vi "Actor Core.vi"(8 "error in":errorcluster, 11 "Pane Settings UI in":refnum<class "Pane Settings UI.lvclass">) -> (0 "error out":errorcluster, 3 "Actor out":refnum<class "Actor.lvclass">)   [LabVIEW 2015, in "Pane Settings UI.lvlib" / "Pane Settings UI.lvclass"]
doc: "The user interface for this panel.\n\n----\nPlease see the following web address for additional documentation and tutorial information:\nhttp://www.mooregoodideas.com/mgi-panel-manager/\n\nAuthor: Derek Trepanier\n\nCopyright (c) 2018, Moore Good Ideas, Inc.\n\nAll rights reserved.\n\nRedistribution and use in source and binary forms, with or without modification, are permitted provided that the following conditions are met:\n\n * Redistributions of source code must retain the above copyright notice, this list of conditions and the following disclaimer.\n * Redistributions in binary form must reproduce the above copyright notice, this list of conditions and the following disclaimer in the documentation and/or other materials provided with the distribution.\n * Neither the name of Moore Good Ideas, Inc. nor the names of its contributors may be used to endorse or promote products derived from this software without specific prior written permission.\n\nTHIS SOFTWARE IS PROVIDED BY THE COPYRIGHT HOLDERS AND CONTRIBUTORS \"AS IS\" AND ANY EXPRESS OR IMPLIED WARRANTIES, INCLUDING, BUT NOT LIMITED TO, THE IMPLIED WARRANTIES OF MERCHANTABILITY AND FITNESS FOR A PARTICULAR PURPOSE ARE DISCLAIMED. IN NO EVENT SHALL THE COPYRIGHT OWNER OR CONTRIBUTORS BE LIABLE FOR ANY DIRECT, INDIRECT, INCIDENTAL, SPECIAL, EXEMPLARY, OR CONSEQUENTIAL DAMAGES (INCLUDING, BUT NOT LIMITED TO, PROCUREMENT OF SUBSTITUTE GOODS OR SERVICES; LOSS OF USE, DATA, OR PROFITS; OR BUSINESS INTERRUPTION) HOWEVER CAUSED AND ON ANY THEORY OF LIABILITY, WHETHER IN CONTRACT, STRICT LIABILITY, OR TORT (INCLUDING NEGLIGENCE OR OTHERWISE) ARISING IN ANY WAY OUT OF THE USE OF THIS SOFTWARE, EVEN IF ADVISED OF THE POSSIBILITY OF SUCH DAMAGE."
uses:
  Pane Settings UI.lvclass
  <vilib>/ActorFramework/Actor/Actor.lvclass
  Typedefs/Point--Cluster.ctl
  Typedefs/Scrollbar Visibility--Enum.ctl
  Classes/Pane/Pane.lvclass
  <vilib>/ActorFramework/Actor/Actor.lvclass/Actor.ctl
  Pane Settings UI.lvclass/Pane Settings UI.ctl
  <vilib>/ActorFramework/Message Enqueuer/Message Enqueuer.lvclass/Message Enqueuer.ctl
  <vilib>/ActorFramework/Message Enqueuer/Enqueue.vi
  <vilib>/ActorFramework/Message Priority Queue/Priority Enqueue.vi
  Pane Relief Main UI/Pane Relief Main UI Messages/Panel Object Settings Changed Msg/Panel Object Settings Changed Msg.lvclass
  <vilib>/MGI/Panel Manager/Panel Actor/Panel Actor/Panel Actor.lvclass
panel:
  in  "Label":string
  in  "Set Min to Current":bool
  in  "Vertical Scroll":T1
  in  "Horizontal Scroll":T1 caption="Scrollbar"
  in  "Origin":T2
  in  "Min Pane":T2={"Horizontal"=1, "Vertical"=0} {"Vertical" min=0; "Horizontal" min=1}
  in  "Color":u32(colorbox)
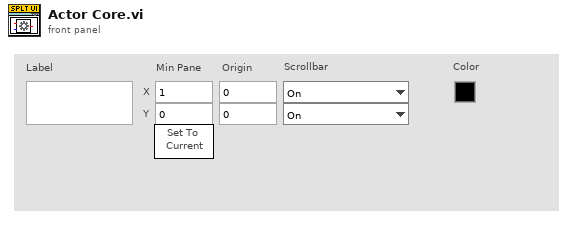
[diagram p1: front panel]
types:
  T1 = typedef "Scrollbar Visibility--Enum.ctl" = enum16{"On", "Off", "Off While Running"}
  T2 = typedef "Point--Cluster.ctl" = cluster{"Horizontal":i32, "Vertical":i32}
  T3 = cluster{"Event Registration Refnum":refnum<event-registration>, "Pnl Actor":refnum<event-registration>}
  T4 = typedef "LVPointTypeDef.ctl" = cluster{"Horizontal":i16, "Vertical":i16}
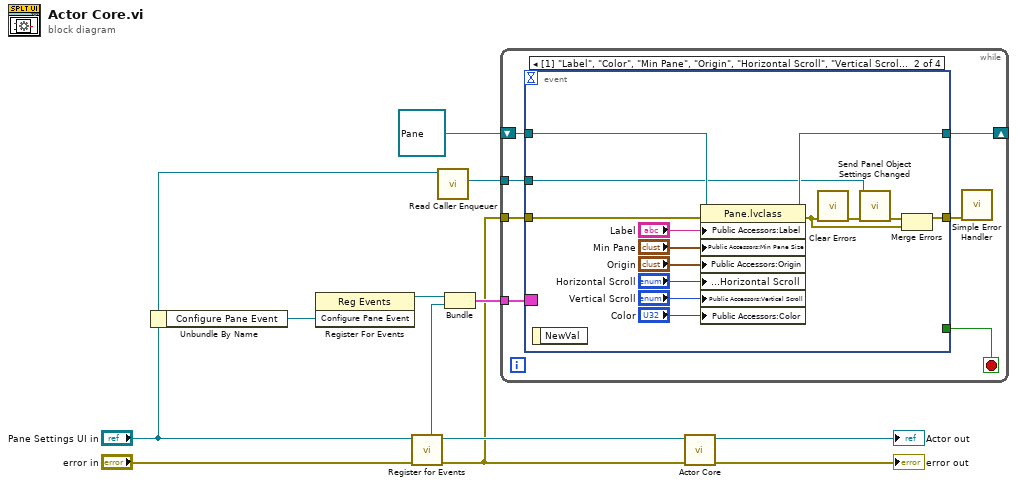
[diagram p0: block diagram]
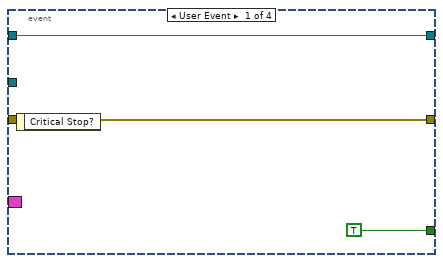
[diagram p2: hidden frame]
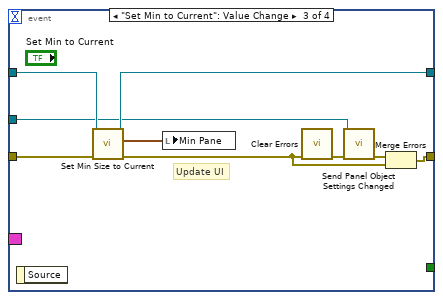
[diagram p3: hidden frame]
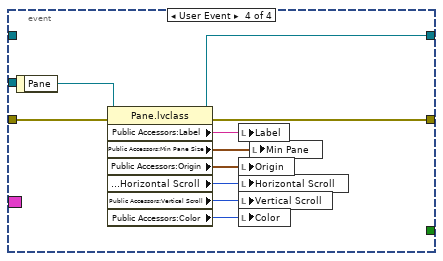
[diagram p4: hidden frame]
diagram:
  n1 = Unbundle By Name("Pane Settings UI in") -> ("Configure Pane Event"=w1:refnum<user-event>)
  n2 = register-events(w1) -> (reference out=w8:refnum<event-registration>)  [unwired: 2 in, 1 out]
  n3 = call <vilib>:"Register for Events.vi"("Error In"="error in", "Panel Actor in"="Pane Settings UI in") -> ("Error Out"=w4:errorcluster, "Panel Actor out"=w10:refnum<class "Pane Settings UI.lvclass">, "Pnl Actor"=w7:refnum<event-registration>)  [unwired: 6 in, 1 out]
  n4 = call <vilib>:"Read Caller Enqueuer.vi"("Actor"="Pane Settings UI in") -> ("Caller Enqueuer"=w3:refnum<class "Message Enqueuer.lvclass">)  [unwired: 10 in]
  n5 = Bundle("Event Registration Refnum"=w8, "Pnl Actor"=w7) -> (w6:T3)  [unwired: 1 in]
  n6 = while {
    tunnel: w6 -> [w19]
    shift-right: [w17] -> _
    shift-left: refnum<class "Pane.lvclass"> refnum ("Pane.lvclass") -> [w16]
    tunnel: w3 -> [w14]
    tunnel: w4 -> [w15]
    stop <- w18 stop-if-true
    n7 = event shown="[1] \"Label\", \"Color\", \"Min Pane\", \"Origin\", \"Horizontal Scroll\", \"Vertical Scroll\": Value Change" {
      selector: w19 -> [_ _ _ _]
      dyn-events: _ -> [_ _ _ _]
      timeout: _ -> [_ _ _ _]
      tunnel: [TRUE _ _ _] -> w18
      tunnel: [w21 w29 w43 w53] -> w17
      tunnel: w16 -> [w21 w28 w44 _]
      tunnel: w15 -> [w20 w36 w45 w55]
      tunnel: [w20 w25 w38 w54] -> w13
      tunnel: w14 -> [_ w23 w37 _]
      event User Event {
        n8 = event-data() -> ()  [unwired: 1 in, 1 out]
      }
      event "Label", "Color": Value Change {
        n9 = event-data() -> ()  [unwired: 1 in, 1 out]
        n10 = property class="Pane.lvclass"(reference=w28, error in=w36, "Public Accessors:Label"="Label", "Public Accessors:Min Pane Size"="Min Pane", "Public Accessors:Origin"="Origin", "Public Accessors:Horizontal Scroll"="Horizontal Scroll", "Public Accessors:Vertical Scroll"="Vertical Scroll", "Public Accessors:Color"="Color") -> (reference out=w29:refnum<class "Pane.lvclass">, error out=w24:errorcluster)
        n11 = call <vilib>:"Clear Errors.vi"("error in (no error)"=w24) -> ("error out"=w27:errorcluster)  [unwired: 5 in, 1 out]
        n12 = call "Send Panel Object Settings Changed.vi"("error in (no error)"=w27, "Message Enqueuer"=w23) -> ("error out"=w26:errorcluster)  [unwired: 8 in, 1 out]
        n13 = Merge Errors(w26, w24) -> (w25:errorcluster)
      }
      event "Set Min to Current": Value Change {
        # "Update UI"
        n14 = event-data() -> ()  [unwired: 1 in, 1 out]
        n15 = call "Set Min Size to Current.vi"("error in (no error)"=w45, "Pane in"=w44) -> ("error out"=w39:errorcluster, "Min Pane Size"=w42:T4, "Pane out"=w43:refnum<class "Pane.lvclass">)  [unwired: 7 in]
        n16 = local write "Min Pane"(w42) -> ()
        n17 = call <vilib>:"Clear Errors.vi"("error in (no error)"=w39) -> ("error out"=w41:errorcluster)  [unwired: 5 in, 1 out]
        n18 = call "Send Panel Object Settings Changed.vi"("error in (no error)"=w41, "Message Enqueuer"=w37) -> ("error out"=w40:errorcluster)  [unwired: 8 in, 1 out]
        n19 = Merge Errors(w40, w39) -> (w38:errorcluster)
      }
      event User Event {
        n20 = event-data() -> ("Pane"=w46:refnum<class "Pane.lvclass">)  [unwired: 1 in]
        n21 = property class="Pane.lvclass"(reference=w46, error in=w55) -> (reference out=w53:refnum<class "Pane.lvclass">, error out=w54:errorcluster, "Public Accessors:Label"=w52:string, "Public Accessors:Min Pane Size"=w51:T2, "Public Accessors:Origin"=w50:T2, "Public Accessors:Horizontal Scroll"=w49:T1, "Public Accessors:Vertical Scroll"=w48:T1, "Public Accessors:Color"=w47:u32)
        n22 = local write "Label"(w52) -> ()
        n23 = local write "Origin"(w50) -> ()
        n24 = local write "Horizontal Scroll"(w49) -> ()
        n25 = local write "Vertical Scroll"(w48) -> ()
        n26 = local write "Color"(w47) -> ()
        n27 = local write "Min Pane"(w51) -> ()
      }
    }
    n28 = call <vilib>:"Simple Error Handler.vi"("error in (no error)"=w13) -> ()  [unwired: 4 in, 5 out]
  }
  n29 = call-parent "Actor Core.vi"("error in"=w4, "Panel Actor in"=w10) -> ("error out"=→"error out":errorcluster, "Actor out"=→"Actor out":refnum<class "Actor.lvclass">)  [unwired: 8 in]
